vi "Initialize.vi"(7 "timeout, ms (5000)":u32=5000, 8 "error in (no error)":errorcluster, 11 "port":refnum<visa-resource-name>) -> (0 "error out":errorcluster, 3 "Arinst SSA-TG out":refnum<class "PL Arinst SSA-TG.lvclass">)   [LabVIEW 2015, in "PL Arinst SSA-TG.lvclass"]
doc: "Initializes connection to device using specified settings."
uses:
  PL Arinst SSA-TG.lvclass
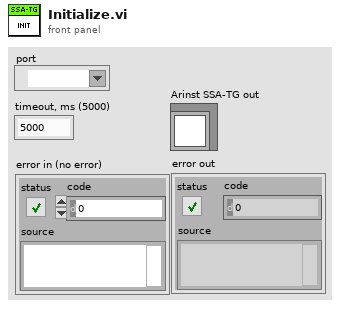
[diagram p1: front panel]
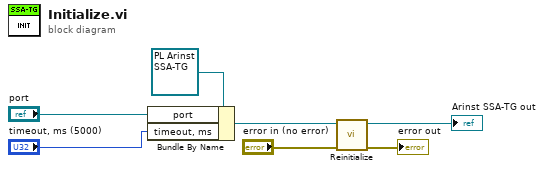
[diagram p0: block diagram]
diagram:
  n1 = Bundle By Name(cluster=refnum<class "PL Arinst SSA-TG.lvclass"> refnum, "port"="port", "timeout, ms"="timeout, ms (5000)") -> (w7:refnum<class "PL Arinst SSA-TG.lvclass">)
  n2 = call "Reinitialize.vi"("error in (no error)"="error in (no error)", "Arinst SSA-TG in"=w7) -> ("error out"=→"error out":errorcluster, "Arinst SSA-TG out"=→"Arinst SSA-TG out":refnum<class "PL Arinst SSA-TG.lvclass">)  [unwired: 8 in]
